vi "신호등.vi"() -> ()   [LabVIEW 2018]
uses:
  TypeDefine/ENUM_TYPE.ctl
panel:
  out "남쪽행 좌회전":cluster{bool, bool, bool}
  out "동쪽행 좌회전":cluster{bool, bool, bool}
  out "서쪽행 좌회전":cluster{bool, bool, bool}
  out "북쪽행 좌회전":cluster{bool, bool, bool}
  in  "동쪽 좌회전 센서":bool
  in  "남쪽 좌회전 센서":bool
  in  "북쪽 좌회전 센서":bool
  in  "서쪽 좌회전 센서":bool
  in  "정지":bool
  out "북쪽행":cluster{bool, bool, bool}
  out "동쪽행":cluster{bool, bool, bool}
  out "서쪽행":cluster{bool, bool, bool}
  out "남쪽행":cluster{bool, bool, bool}
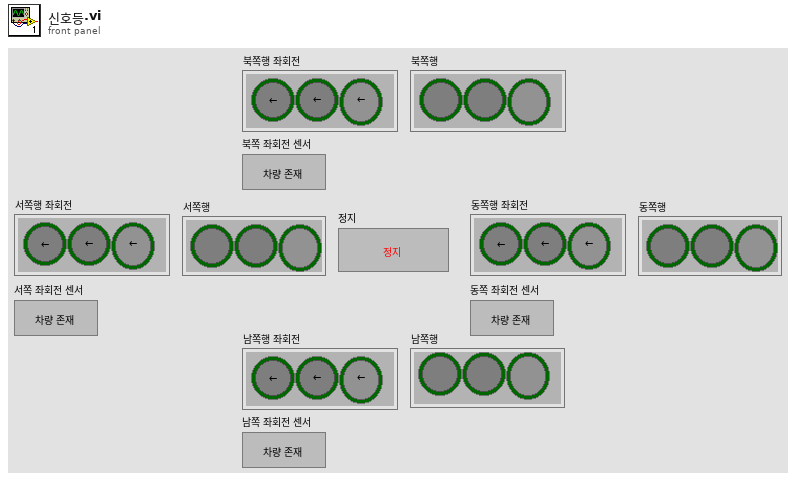
[diagram p1: front panel]
types:
  T1 = typedef "ENUM_TYPE.ctl" = enum16{"북남초", "북남노", "동서초", "동서노", "초기화", "정지", "북남센", "동서센", "북남좌", "동서좌", "북남좌노", "동서좌노"}
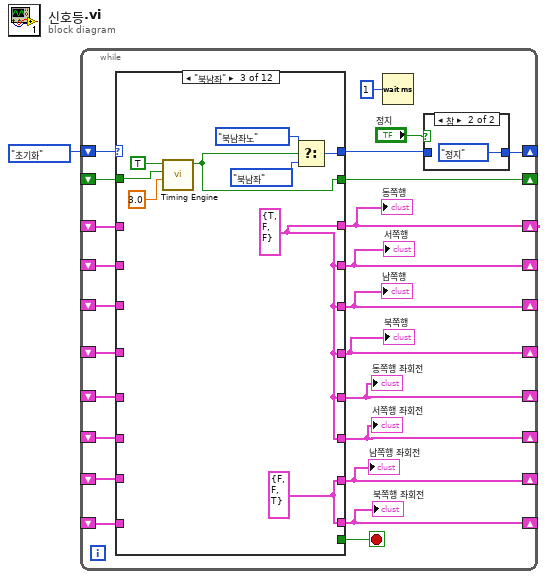
[diagram p0: block diagram]
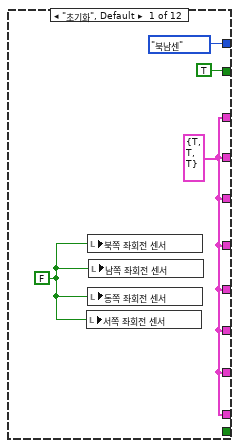
[diagram p3: hidden frame]
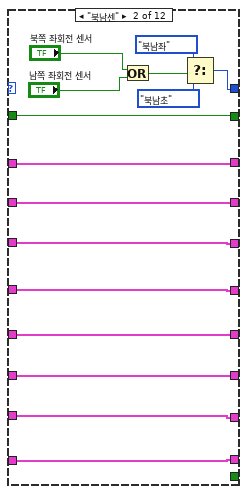
[diagram p4: hidden frame]
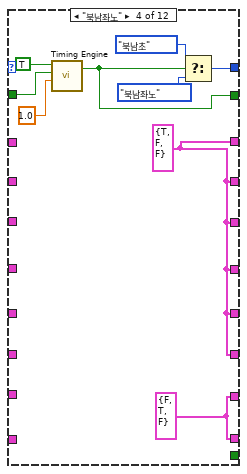
[diagram p5: hidden frame]
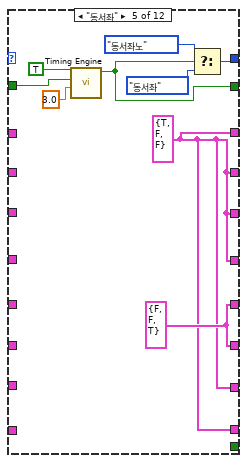
[diagram p6: hidden frame]
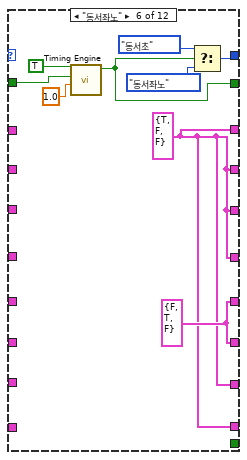
[diagram p7: hidden frame]
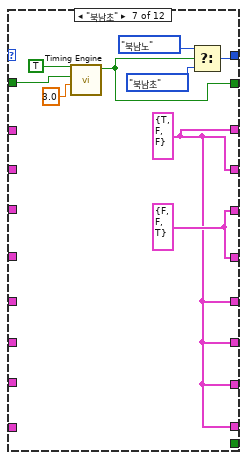
[diagram p8: hidden frame]
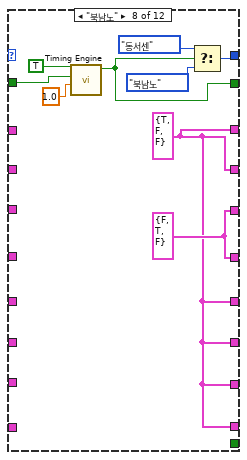
[diagram p9: hidden frame]
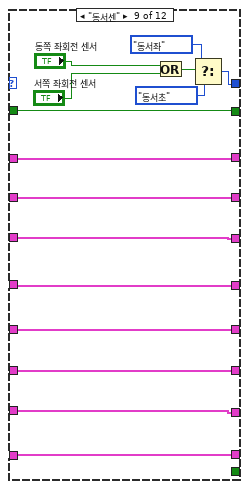
[diagram p10: hidden frame]
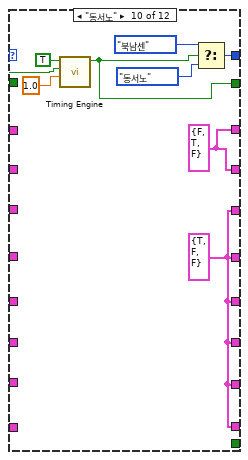
[diagram p11: hidden frame]
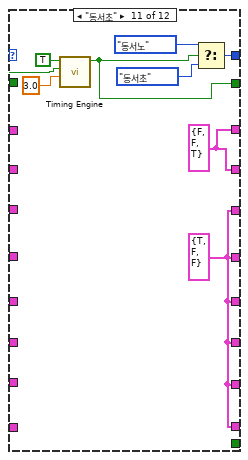
[diagram p12: hidden frame]
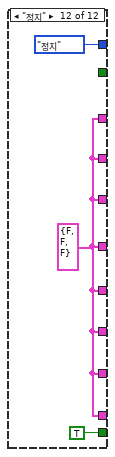
[diagram p13: hidden frame]
diagram:
  n1 = while {
    shift-right: [w21] -> _
    shift-left: ENUM_TYPE."초기화" ("열거형") -> [w25]
    shift-right: [w19] -> _
    shift-left: _ -> [w20]
    shift-right: [w17] -> _
    shift-left: _ -> [w2]
    shift-right: [w16] -> _
    shift-left: _ -> [w3]
    shift-right: [w15] -> _
    shift-left: _ -> [w14]
    shift-right: [w4] -> _
    shift-left: _ -> [w13]
    shift-right: [w12] -> _
    shift-left: _ -> [w11]
    shift-right: [w10] -> _
    shift-left: _ -> [w9]
    shift-right: [w8] -> _
    shift-left: _ -> [w7]
    shift-right: [w6] -> _
    shift-left: _ -> [w5]
    stop <- w24 stop-if-true
    n2 = case shown="\"북남좌\"" w25 {
      tunnel: [ENUM_TYPE."북남센" ("열거형") w45 w54 w63 w72 w81 w90 w99 w114 w122 w131 ENUM_TYPE."정지" ("열거형")] -> w22
      tunnel: [w31 w35 w47 w57 w65 w74 w83 w92 w102 w124 w133 w135] -> w17
      tunnel: [w31 w34 w47 w57 w65 w74 w83 w92 w103 w124 w133 w135] -> w16
      tunnel: [w31 w42 w47 w57 w65 w74 w84 w93 w110 w118 w127 w135] -> w15
      tunnel: [w31 w41 w47 w57 w65 w74 w84 w93 w109 w118 w127 w135] -> w4
      tunnel: [_ _ _ _ _ _ _ _ _ _ _ TRUE] -> w24
      tunnel: w20 -> [_ w36 w53 w62 w71 w80 w89 w98 w104 w120 w129 _]
      tunnel: [TRUE w36 w49 w56 w67 w76 w85 w94 w104 w119 w128 _] -> w19
      tunnel: [w31 w40 w47 w57 w66 w75 w83 w92 w108 w118 w127 w135] -> w12
      tunnel: [w31 w39 w47 w57 w66 w75 w83 w92 w107 w118 w127 w135] -> w10
      tunnel: [w31 w38 w48 w58 w65 w74 w83 w92 w106 w118 w127 w135] -> w8
      tunnel: [w31 w37 w48 w58 w65 w74 w83 w92 w105 w118 w127 w135] -> w6
      tunnel: w14 -> [_ w42 _ _ _ _ _ _ w110 _ _ _]
      tunnel: w13 -> [_ w41 _ _ _ _ _ _ w109 _ _ _]
      tunnel: w11 -> [_ w40 _ _ _ _ _ _ w108 _ _ _]
      tunnel: w9 -> [_ w39 _ _ _ _ _ _ w107 _ _ _]
      tunnel: w7 -> [_ w38 _ _ _ _ _ _ w106 _ _ _]
      tunnel: w5 -> [_ w37 _ _ _ _ _ _ w105 _ _ _]
      tunnel: w3 -> [_ w34 _ _ _ _ _ _ w103 _ _ _]
      tunnel: w2 -> [_ w35 _ _ _ _ _ _ w102 _ _ _]
      frame "초기화", Default {
        w29 = FALSE
        w31 = cluster{bool, bool, bool} {TRUE, TRUE, TRUE} ("북쪽행")
        n3 = local write "서쪽 좌회전 센서"(w29) -> ()
        n4 = local write "북쪽 좌회전 센서"(w29) -> ()
        n5 = local write "동쪽 좌회전 센서"(w29) -> ()
        n6 = local write "남쪽 좌회전 센서"(w29) -> ()
      }
      frame "북남센" {
        n7 = Or(x="북쪽 좌회전 센서", y="남쪽 좌회전 센서") -> (x .or. y?=w46:bool)
        n8 = Select(t=ENUM_TYPE."북남좌" ("열거형"), s=w46, f=ENUM_TYPE."북남초" ("열거형")) -> (s? t:f=w45:T1)
      }
      frame "북남좌" {
        w47 = cluster{bool, bool, bool} {TRUE, FALSE, FALSE} ("북쪽행")
        w48 = cluster{bool, bool, bool} {FALSE, FALSE, TRUE} ("북쪽행")
        n9 = call "Timing Engine.vi"("시간 제한"=3.0, "리셋"=w53, "진행 시간?"=TRUE) -> ("시간 만료됨?"=w49:bool)  [unwired: 1 in, 7 out]
        n10 = Select(t=ENUM_TYPE."북남좌노" ("열거형"), s=w49, f=ENUM_TYPE."북남좌" ("열거형")) -> (s? t:f=w54:T1)
      }
      frame "북남좌노" {
        w57 = cluster{bool, bool, bool} {TRUE, FALSE, FALSE} ("북쪽행")
        w58 = cluster{bool, bool, bool} {FALSE, TRUE, FALSE} ("북쪽행")
        n11 = call "Timing Engine.vi"("시간 제한"=1.0, "리셋"=w62, "진행 시간?"=TRUE) -> ("시간 만료됨?"=w56:bool)  [unwired: 1 in, 7 out]
        n12 = Select(t=ENUM_TYPE."북남초" ("열거형"), s=w56, f=ENUM_TYPE."북남좌노" ("열거형")) -> (s? t:f=w63:T1)
      }
      frame "동서좌" {
        w65 = cluster{bool, bool, bool} {TRUE, FALSE, FALSE} ("북쪽행")
        w66 = cluster{bool, bool, bool} {FALSE, FALSE, TRUE} ("북쪽행")
        n13 = call "Timing Engine.vi"("시간 제한"=3.0, "리셋"=w71, "진행 시간?"=TRUE) -> ("시간 만료됨?"=w67:bool)  [unwired: 1 in, 7 out]
        n14 = Select(t=ENUM_TYPE."동서좌노" ("열거형"), s=w67, f=ENUM_TYPE."동서좌" ("열거형")) -> (s? t:f=w72:T1)
      }
      frame "동서좌노" {
        w74 = cluster{bool, bool, bool} {TRUE, FALSE, FALSE} ("북쪽행")
        w75 = cluster{bool, bool, bool} {FALSE, TRUE, FALSE} ("북쪽행")
        n15 = call "Timing Engine.vi"("시간 제한"=1.0, "리셋"=w80, "진행 시간?"=TRUE) -> ("시간 만료됨?"=w76:bool)  [unwired: 1 in, 7 out]
        n16 = Select(t=ENUM_TYPE."동서초" ("열거형"), s=w76, f=ENUM_TYPE."동서좌노" ("열거형")) -> (s? t:f=w81:T1)
      }
      frame "북남초" {
        w83 = cluster{bool, bool, bool} {TRUE, FALSE, FALSE} ("북쪽행")
        w84 = cluster{bool, bool, bool} {FALSE, FALSE, TRUE} ("북쪽행")
        n17 = call "Timing Engine.vi"("시간 제한"=3.0, "리셋"=w89, "진행 시간?"=TRUE) -> ("시간 만료됨?"=w85:bool)  [unwired: 1 in, 7 out]
        n18 = Select(t=ENUM_TYPE."북남노" ("열거형"), s=w85, f=ENUM_TYPE."북남초" ("열거형")) -> (s? t:f=w90:T1)
      }
      frame "북남노" {
        w92 = cluster{bool, bool, bool} {TRUE, FALSE, FALSE} ("북쪽행")
        w93 = cluster{bool, bool, bool} {FALSE, TRUE, FALSE} ("북쪽행")
        n19 = call "Timing Engine.vi"("시간 제한"=1.0, "리셋"=w98, "진행 시간?"=TRUE) -> ("시간 만료됨?"=w94:bool)  [unwired: 1 in, 7 out]
        n20 = Select(t=ENUM_TYPE."동서센" ("열거형"), s=w94, f=ENUM_TYPE."북남노" ("열거형")) -> (s? t:f=w99:T1)
      }
      frame "동서센" {
        n21 = Or(x="동쪽 좌회전 센서", y="서쪽 좌회전 센서") -> (x .or. y?=w115:bool)
        n22 = Select(t=ENUM_TYPE."동서좌" ("열거형"), s=w115, f=ENUM_TYPE."동서초" ("열거형")) -> (s? t:f=w114:T1)
      }
      frame "동서노" {
        w124 = cluster{bool, bool, bool} {FALSE, TRUE, FALSE} ("북쪽행")
        w118 = cluster{bool, bool, bool} {TRUE, FALSE, FALSE} ("북쪽행")
        n23 = call "Timing Engine.vi"("시간 제한"=1.0, "리셋"=w120, "진행 시간?"=TRUE) -> ("시간 만료됨?"=w119:bool)  [unwired: 1 in, 7 out]
        n24 = Select(t=ENUM_TYPE."북남센" ("열거형"), s=w119, f=ENUM_TYPE."동서노" ("열거형")) -> (s? t:f=w122:T1)
      }
      frame "동서초" {
        w133 = cluster{bool, bool, bool} {FALSE, FALSE, TRUE} ("북쪽행")
        w127 = cluster{bool, bool, bool} {TRUE, FALSE, FALSE} ("북쪽행")
        n25 = call "Timing Engine.vi"("시간 제한"=3.0, "리셋"=w129, "진행 시간?"=TRUE) -> ("시간 만료됨?"=w128:bool)  [unwired: 1 in, 7 out]
        n26 = Select(t=ENUM_TYPE."동서노" ("열거형"), s=w128, f=ENUM_TYPE."동서초" ("열거형")) -> (s? t:f=w131:T1)
      }
      frame "정지" {
        w135 = cluster{bool, bool, bool} {FALSE, FALSE, FALSE} ("북쪽행")
      }
    }
    "동쪽행" <- w17
    "서쪽행" <- w16
    "남쪽행" <- w15
    "북쪽행" <- w4
    "남쪽행 좌회전" <- w8
    "동쪽행 좌회전" <- w12
    "서쪽행 좌회전" <- w10
    "북쪽행 좌회전" <- w6
    n27 = Wait (ms)(milliseconds to wait=u32 1 ("대기 시간 (ms)")) -> ()  [unwired: 1 out]
    n28 = case shown="참" "정지" {
      tunnel: w22 -> [w26 _]
      tunnel: [w26 ENUM_TYPE."정지" ("열거형")] -> w21
      frame False {
      }
      frame True {
      }
    }
  }
